vi "DriveGetSpeedModifer.vi"() -> (3 "SpeedModifer":dbl)   [LabVIEW 2020]
uses:
  DriveGlobal.vi
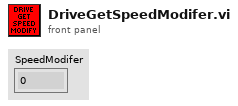
[diagram p1: front panel]
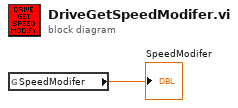
[diagram p0: block diagram]
diagram:
  n1 = global read "DriveGlobal.vi" "SpeedModifer"() -> (→"SpeedModifer":dbl)
